vi "Simulator for Automatic water level.vi"() -> ()   [LabVIEW 2016]
panel:
  out "Lower Tank ultrasonic Sensor reading":dbl
  out "Upper Tank Ultrasonic sensor  reading":dbl
  in  "Lower Tank starting level":dbl
  in  "Upper Tank Starting Level":dbl
  in  "Upper Required Level":dbl
  out "Lower Tank":dbl(slide) scale=0.0..35.0
  out "Upper Tank":dbl(slide) scale=0.0..35.0
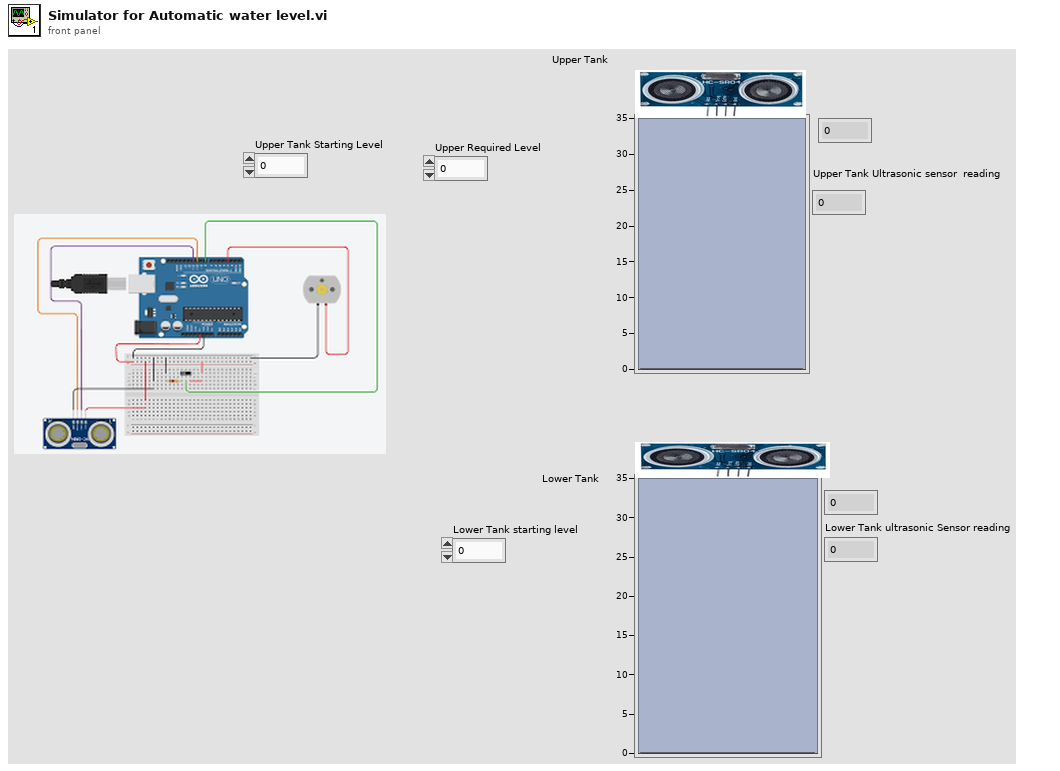
[diagram p1: front panel]
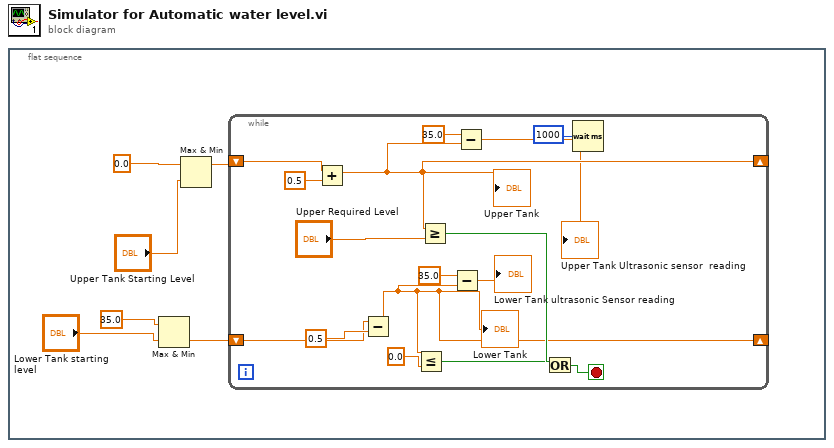
[diagram p0: block diagram]
diagram:
  n1 = flat-sequence {
    frame #0 {
      n2 = Max & Min(x=35.0 ("x-y"), y="Lower Tank starting level") -> (min(x,y)=w2:dbl)  [unwired: 1 out]
      n3 = Max & Min(x=0.0, y="Upper Tank Starting Level") -> (max(x,y)=w5:dbl)  [unwired: 1 out]
      n4 = while {
        shift-right: [w12] -> _
        shift-left: w5 -> [w20]
        shift-right: [w9] -> _
        shift-left: w2 -> [w17]
        stop <- w16 stop-if-true
        n5 = Add(x=w20, y=0.5) -> (x+y=w12:dbl)
        "Upper Tank" <- w12
        n6 = Subtract(x=w17, y=0.5) -> (x-y=w9:dbl)
        "Lower Tank" <- w9
        n7 = Less Or Equal?(x=w9, y=0.0 ("x")) -> (x <= y?=w14:bool)
        n8 = Greater Or Equal?(x=w12, y="Upper Required Level") -> (x >= y?=w15:bool)
        n9 = Subtract(x=35.0, y=w9) -> (x-y=→"Lower Tank ultrasonic Sensor reading":dbl)
        n10 = Subtract(x=35.0, y=w12) -> (x-y=→"Upper Tank Ultrasonic sensor  reading":dbl)
        n11 = Or(x=w15, y=w14) -> (x .or. y?=w16:bool)
        n12 = Wait (ms)(milliseconds to wait=u32 1000) -> ()  [unwired: 1 out]
      }
    }
  }
